vi "process.vi"(8 "error in":errorcluster, 10 "responder in":refnum<class "http responder.lvclass">, 11 "Basic HTTP server in":refnum<class "Basic HTTP server.lvclass">) -> (0 "error out":errorcluster, 2 "responder out":refnum<class "http responder.lvclass">, 3 "Basic HTTP server out":refnum<class "Basic HTTP server.lvclass">)   [LabVIEW 2013, in "Basic HTTP server.lvclass"]
uses:
  Basic HTTP server.lvclass
  HTTP responder/http responder.lvclass
  Basic HTTP server.lvclass/Basic HTTP server.ctl
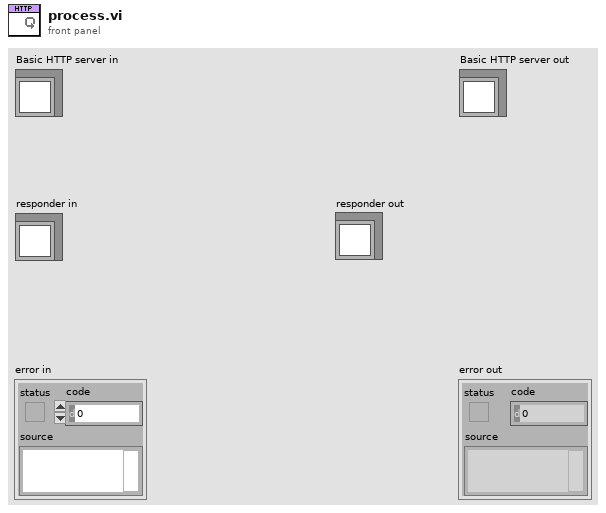
[diagram p1: front panel]
types:
  T1 = typedef "Basic HTTP server.lvclass/http server properties.ctl" = cluster{"max url size":i32, "max header":i32, "timeout ms":i32, "max data size":i32}
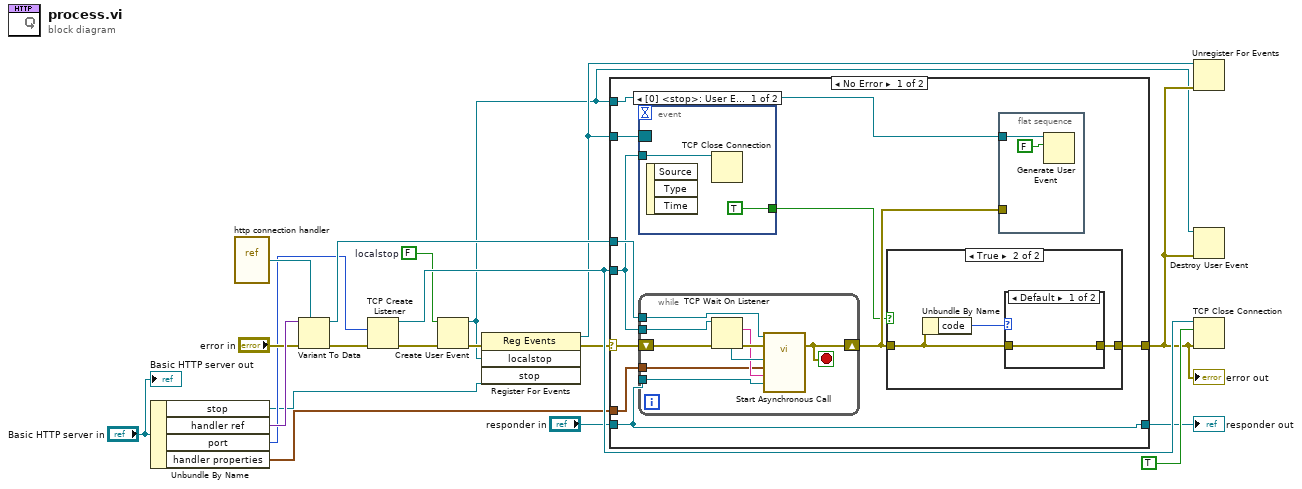
[diagram p0: block diagram]
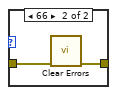
[diagram p3: hidden frame]
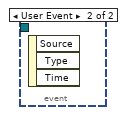
[diagram p4: hidden frame]
diagram:
  w3 = FALSE  # localstop
  n1 = Unbundle By Name("Basic HTTP server in") -> ("stop"=w6:refnum<user-event>, "handler ref"=w17:variant, "port"=w12:u16, "handler properties"=w11:T1)
  n2 = vi-ref "http connection handler.vi"() -> (w16:refnum<vi>)
  n3 = Variant To Data(error in="error in", type=w16, Variant=w17) -> (data=w14:refnum<vi>, error out=w13:errorcluster)
  n4 = TCP Create Listener(8:w13, 10:w12) -> (0:w9:errorcluster, 3:w20:refnum<k5>)  [unwired: 3 in, 1 out]
  n5 = Create User Event(user event datatype=w3, error in=w9) -> (user event=w1:refnum<user-event>, error out=w4:errorcluster)
  n6 = register-events(error in=w4, w1, w6) -> (reference out=w5:refnum<event-registration>, error out=w7:errorcluster)  [unwired: 1 in]
  n7 = case shown="No Error" w7 {
    selector: w7 -> [w30 w52]
    tunnel: [w22 w52] -> w2
    tunnel: w20 -> [w26 _]
    tunnel: w14 -> [w29 _]
    tunnel: w11 -> [w28 _]
    tunnel: "responder in" -> [w27 w51]
    tunnel: [w27 w51] -> w8
    tunnel: w5 -> [w25 _]
    tunnel: w1 -> [w24 _]
    frame No Error {
      n8 = event shown="[0] <stop>: User Event" {
        selector: w25 -> [_ _]
        dyn-events: _ -> [_ _]
        timeout: _ -> [_ _]
        tunnel: w26 -> [w41 _]
        tunnel: [TRUE _] -> w21
        event User Event {
          n9 = event-data() -> ()  [unwired: 1 in, 3 out]
          n10 = TCP Close Connection(connection ID=w41) -> ()  [unwired: 2 in, 2 out]
        }
        event User Event {
          n11 = event-data() -> ()  [unwired: 1 in, 3 out]
        }
      }
      n12 = while {
        shift-right: [w47] -> w23
        shift-left: w30 -> [w50]
        tunnel: w26 -> [w49]
        tunnel: w29 -> [w46]
        tunnel: w28 -> [w43]
        tunnel: w27 -> [w42]
        stop <- w47 stop-if-true
        n13 = TCP Wait On Listener(8:w50, 11:w49) -> (0:w48:errorcluster, 2:w44:string, 4:w45:refnum<k5>)  [unwired: 2 in, 2 out]
        n14 = call-by-ref "Start Asynchronous Call"(reference=w46, error in=w48, "http responder"=w42, "remote address"=w44, "server properties"=w43, "connection"=w45) -> (error out=w47:errorcluster)  [unwired: 8 in, 1 out]
      }
      n15 = case shown="True" w21 {
        tunnel: w23 -> [w31 w33]
        tunnel: [w31 w34] -> w22
        frame False {
        }
        frame True {
          n16 = Unbundle By Name(w33) -> ("code"=w32:i32)
          n17 = case shown="Default" w32 {
            tunnel: w33 -> [w35 w37]
            tunnel: [w35 w36] -> w34
            frame Default {
            }
            frame 66 {
              n18 = call <vilib>:"Clear Errors.vi"("error in (no error)"=w37) -> ("error out"=w36:errorcluster)  [unwired: 6 in]
            }
          }
        }
      }
      n19 = flat-sequence {
        tunnel: w23 -> [_]
        tunnel: w24 -> [w39]
        frame #0 {
          n20 = Generate User Event(user event=w39, event data cluster=FALSE ("event data")) -> ()  [unwired: 2 in, 2 out]
        }
      }
    }
    frame Error {
    }
  }
  "error out" <- w2
  "responder out" <- w8
  n21 = Unregister For Events(event registration refnum=w5, error in=w2) -> ()  [unwired: 1 out]
  n22 = Destroy User Event(user event=w1, error in=w2) -> ()  [unwired: 1 out]
  n23 = TCP Close Connection(connection ID=w20, abort (F)=TRUE, error in (no error)=w2) -> ()  [unwired: 2 out]
  "Basic HTTP server out" <- "Basic HTTP server in"
